vi "Drive Base Immediate Wrapper.vi"() -> ()   [LabVIEW 2019]
uses:
  Implementation/Drive Base Operations.ctl
panel:
  in  "Synchronication":enum16{"Start", "Wait"}(ring)
  in  "Right Setpoint":dbl
  in  "Left Setpoint":dbl
  in  "Operation":T1
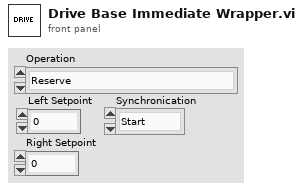
[diagram p1: front panel]
types:
  T1 = typedef "Drive Base Operations.ctl" = enum16{"Reserve", "Read Current", "Immediate", "Limelight", "Manual Adjustment", "Limelight + Shoot", "Play Path"}
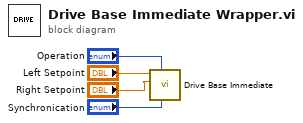
[diagram p0: block diagram]
diagram:
  n1 = call "Drive Base Immediate.vi"("Synchronication"="Synchronication", "Operation"="Operation", "Right Setpoint"="Right Setpoint", "Left Setpoint"="Left Setpoint") -> ()  [unwired: 7 in, 1 out]
